vi "Encode_SignedHundredths.vi"(1 "Signed Hundredths (0.00)":dbl[](array[numeric])) -> (0 "Little Endian":u8[](array[numeric]))   [LabVIEW 2015, in "navX Library v3.lvlib" / "navX Registry Cache.lvclass"]
uses:
  navX Registry Cache.lvclass
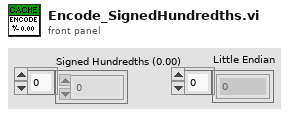
[diagram p1: front panel]
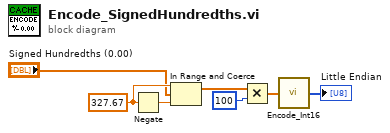
[diagram p0: block diagram]
diagram:
  w7 = 327.67
  n1 = Negate(x=w7) -> (-x=w6:dbl)
  n2 = In Range and Coerce(upper limit=w7, x="Signed Hundredths (0.00)", lower limit=w6) -> (coerced(x)=w3:dbl[])  [unwired: 1 out]
  n3 = Multiply(x=w3, y=100) -> (x*y=w2:dbl[])
  n4 = call "Encode_Int16.vi"("Int16"=w2) -> ("Little Endian"=→"Little Endian":u8[])
